vi "SDSU_MemWrite.vi"(6 "board dest":i32, 8 "error in (no error)":errorcluster, 9 "type":string, 10 "args":string, 11 "fd":i32) -> (0 "error out":errorcluster, 2 "return value":i32, 3 "fd out":i32)   [LabVIEW 2016]
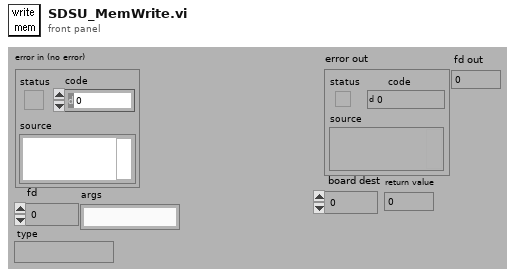
[diagram p1: front panel]
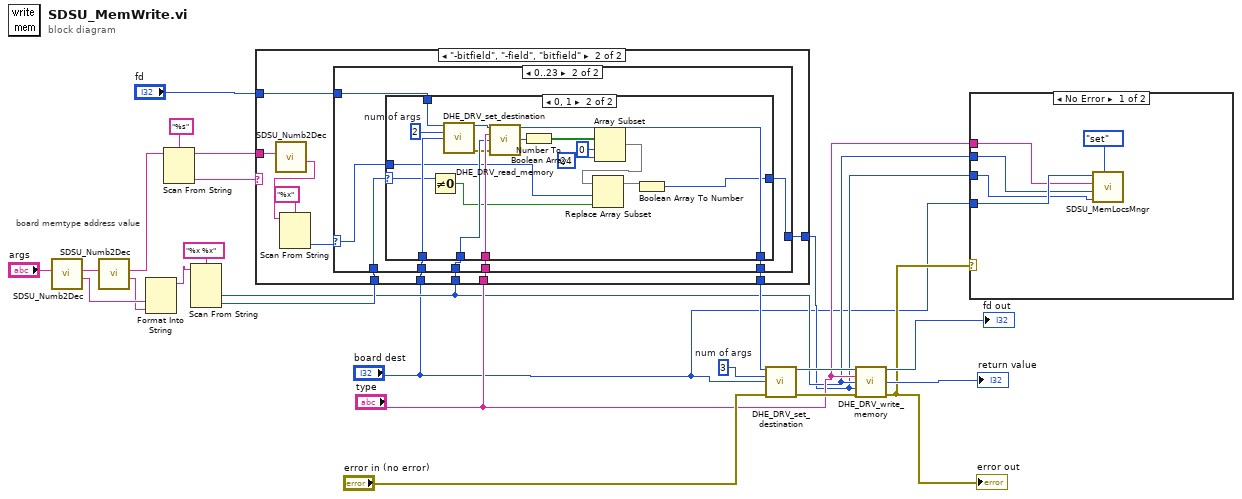
[diagram p0: block diagram]
diagram:
  w24 = 3  # num of args
  # "board memtype address value"
  n1 = call "SDSU_Numb2Dec.vi"("input str"="args") -> ("output hexa"=w18:string, "remaining string"=w19:string)  [unwired: 9 out]
  n2 = call "SDSU_Numb2Dec.vi"("input str"=w19) -> ("output hexa"=w17:string, "remaining string"=w9:string)  [unwired: 9 out]
  n3 = Format Into String(w18, w17) -> (resulting string=w16:string)  [unwired: 3 in, 1 out]
  n4 = Scan From String(format string="%s", input string=w9) -> (remaining string=w6:string, output 1=w8:string)  [unwired: 2 in, 3 out]
  n5 = Scan From String(format string="%x %x" ("Format String"), input string=w16) -> (output 1=w3:u32, output 2=w12:u32)  [unwired: 2 in, 5 out]
  n6 = case shown="\"-bitfield\", \"-field\", \"bitfield\"" w8 {
    tunnel: w12 -> [w26 w32]
    tunnel: [w26 w31] -> w2
    tunnel: "fd" -> [w25 w37]
    tunnel: [w25 w36] -> w10
    tunnel: "type" -> [_ w35]
    tunnel: w3 -> [_ w34]
    tunnel: "board dest" -> [_ w33]
    tunnel: w6 -> [_ w30]
    frame Default {
    }
    frame "-bitfield", "-field", "bitfield" {
      n7 = call "SDSU_Numb2Dec.vi"("input str"=w30) -> ("output hexa"=w29:string)  [unwired: 10 out]
      n8 = Scan From String(format string="%x", input string=w29) -> (output 1=w27:u32)  [unwired: 2 in, 4 out]
      n9 = case shown="0..23" w27 {
        selector: w27 -> [_ w40]
        tunnel: w37 -> [w38 w47]
        tunnel: [w38 w46] -> w36
        tunnel: w35 -> [_ w45]
        tunnel: w34 -> [_ w44]
        tunnel: w33 -> [_ w43]
        tunnel: w32 -> [w39 w42]
        tunnel: [w39 w41] -> w31
        frame Default {
        }
        frame 0..23 {
          n10 = case shown="0, 1" w42 {
            selector: w42 -> [w49 w53]
            tunnel: w47 -> [w48 w65]
            tunnel: [w48 w64] -> w46
            tunnel: w45 -> [_ w63]
            tunnel: w44 -> [_ w62]
            tunnel: w43 -> [_ w61]
            tunnel: [w49 w50] -> w41
            tunnel: w40 -> [_ w55]
            frame Default {
            }
            frame 0, 1 {
              w66 = 2  # num of args
              n11 = Not Equal To 0?(x=w53) -> (x != 0?=w52:bool)
              n12 = call "DHE_DRV_set_destination.vi"("fd"=w65, "num of args"=w66, "board dest"=w61) -> ("fd out"=w67:i32, "error out"=w60:errorcluster)  [unwired: 1 in, 10 out]
              n13 = call "DHE_DRV_read_memory.vi"("fd"=w67, "type"=w63, "address"=w62, "error in (no error)"=w60) -> ("fd"=w64:i32, "return value"=w59:i32)  [unwired: 10 out]
              n14 = Number To Boolean Array(number=w59) -> (Boolean array=w54:bool[])
              n15 = Array Subset(array=w54, index=0, length=24) -> (w56:bool[])
              n16 = Replace Array Subset(array=w56, new element=w52, index=w55) -> (w51:bool[])
              n17 = Boolean Array To Number(Boolean array=w51) -> (number=w50:u32)
            }
          }
        }
      }
    }
  }
  n18 = call "DHE_DRV_set_destination.vi"("fd"=w10, "num of args"=w24, "board dest"="board dest", "error in (no error)"="error in (no error)") -> ("fd out"=w22:i32, "error out"=w23:errorcluster)  [unwired: 10 out]
  n19 = call "DHE_DRV_write_memory.vi"("fd"=w22, "type"="type", "address"=w3, "value"=w2, "error in (no error)"=w23) -> ("fd out"=→"fd out":i32, "return value"=→"return value":i32, "error out"=w5:errorcluster)  [unwired: 8 out]
  "error out" <- w5
  n20 = case shown="No Error" w5 {
    tunnel: "type" -> [w70 _]
    tunnel: w3 -> [w69 _]
    tunnel: w2 -> [w68 _]
    tunnel: "board dest" -> [w71 _]
    frame No Error {
      n21 = call "SDSU_MemLocsMngr.vi"("action"=enum16{"set", "get", "clear"}."set", "value"=w68, "address"=w69, "type"=w70, "board"=w71) -> ()  [unwired: 5 in, 2 out]
    }
    frame Error {
    }
  }
